vi "Untitled 11 (SubVI).vi"(11 "Reset/Count":bool) -> (3 "f":i32)   [LabVIEW 2023]
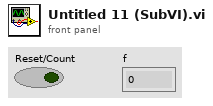
[diagram p1: front panel]
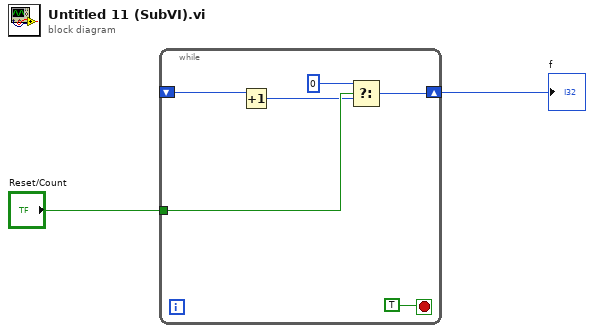
[diagram p0: block diagram]
diagram:
  n1 = while {
    shift-right: [w6] -> w2
    shift-left: _ -> [w7]
    tunnel: "Reset/Count" -> [w5]
    stop <- TRUE stop-if-true
    n2 = Increment(x=w7) -> (x+1=w3:i32)
    n3 = Select(t=0 ("f"), s=w5, f=w3) -> (s? t:f=w6:i32)
  }
  "f" <- w2
